vi "Reserve Session.vi"(6 "contextId":T4, 8 "error in":errorcluster, 9 "timeout (ms)":i32=-1, 10 "Request Data":T5, 11 "gRPC ID":T4) -> (0 "error out":errorcluster, 2 "Session Info":T1, 3 "gRPC ID out":T4)   [LabVIEW 2020]
uses:
  <vilib>/gRPC/LabVIEW gRPC Library/Shared/grpcId.ctl
  <vilib>/MeasurementLink/MeasurementLink Session Management Client/RPC Messages/ni_measurementlink_sessionmanagement_v1_ReserveSessionsRequest.ctl
  <vilib>/MeasurementLink/MeasurementLink Session Management Client/RPC Messages/ni_measurementlink_PinMapContext.ctl
  <vilib>/MeasurementLink/MeasurementLink Session Management Client/RPC Messages/ni_measurementlink_sessionmanagement_v1_SessionInformation.ctl
  <vilib>/MeasurementLink/MeasurementLink Session Management Client/RPC Messages/nidevice_grpc_Session.ctl
  <vilib>/MeasurementLink/MeasurementLink Session Management Client/RPC Messages/ni_measurementlink_sessionmanagement_v1_ChannelMapping.ctl
  <vilib>/MeasurementLink/MeasurementLink Session Management Client/MeasurementLink Session Management Client.lvlib
  <vilib>/gRPC/LabVIEW gRPC Library/grpc-lvsupport-release.lvlib
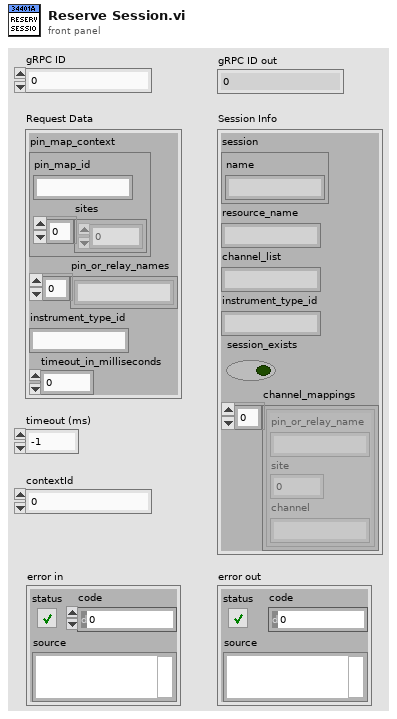
[diagram p1: front panel]
types:
  T1 = typedef "MeasurementLink Session Management Client.lvlib/ni_measurementlink_sessionmanagement_v1_SessionInformation.ctl" = cluster{"session":T2, "resource_name":string, "channel_list":string, "instrument_type_id":string, "session_exists":bool, "channel_mappings":T3[]}
  T2 = typedef "MeasurementLink Session Management Client.lvlib/nidevice_grpc_Session.ctl" = cluster{"name":string}
  T3 = typedef "MeasurementLink Session Management Client.lvlib/ni_measurementlink_sessionmanagement_v1_ChannelMapping.ctl" = cluster{"pin_or_relay_name":string, "site":i32, "channel":string}
  T4 = typedef "grpc-lvsupport-release.lvlib/grpcId.ctl" = u64
  T5 = typedef "MeasurementLink Session Management Client.lvlib/ni_measurementlink_sessionmanagement_v1_ReserveSessionsRequest.ctl" = cluster{"pin_map_context":T6, "pin_or_relay_names":string[], "instrument_type_id":string, "timeout_in_milliseconds":i32}
  T6 = typedef "MeasurementLink Session Management Client.lvlib/ni_measurementlink_PinMapContext.ctl" = cluster{"pin_map_id":string, "sites":i32[]}
  T7 = typedef "MeasurementLink Session Management Client.lvlib/ni_measurementlink_sessionmanagement_v1_ReserveSessionsResponse.ctl" = cluster{"sessions":T1[]}
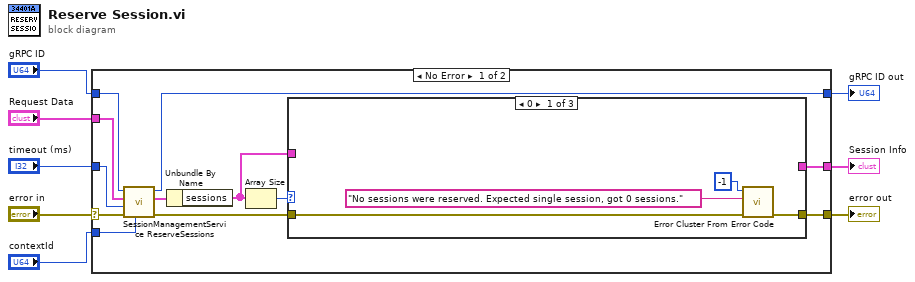
[diagram p0: block diagram]
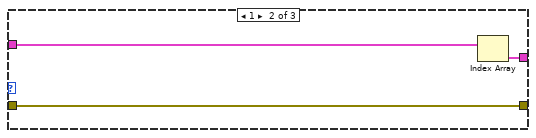
[diagram p2: hidden frame]
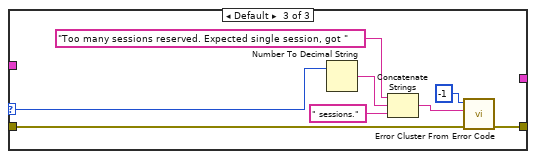
[diagram p3: hidden frame]
diagram:
  n1 = case shown="No Error" "error in" {
    selector: "error in" -> [w16 w36]
    tunnel: [w11 w36] -> w7
    tunnel: "gRPC ID" -> [w15 w37]
    tunnel: [w12 w37] -> w5
    tunnel: "Request Data" -> [w17 _]
    tunnel: "timeout (ms)" -> [w18 _]
    tunnel: "contextId" -> [w14 _]
    tunnel: [w9 _] -> w1
    frame No Error {
      n2 = call <vilib>:"SessionManagementService ReserveSessions.vi"("contextId"=w14, "error in"=w16, "timeout (ms)"=w18, "Request Data"=w17, "gRPC ID"=w15) -> ("error out"=w10:errorcluster, "Response Data"=w13:T7, "gRPC ID out"=w12:T4)  [unwired: 4 in]
      n3 = Unbundle By Name(w13) -> ("sessions"=w19:T1[])
      n4 = Array Size(array=w19) -> (size(s)=w20:i32)
      n5 = case shown="0" w20 {
        selector: w20 -> [_ _ w30]
        tunnel: w10 -> [w24 w25 w35]
        tunnel: [w21 w25 w33] -> w11
        tunnel: w19 -> [_ w27 _]
        tunnel: [_ w26 _] -> w9
        frame 0 {
          n6 = call <vilib>:"Error Cluster From Error Code.vi"("error in (no error)"=w24, "error message (\"\")"="No sessions were reserved. Expected single session, got 0 sessions." ("error message (\"\")"), "error code (0)"=-1) -> ("error out"=w21:errorcluster)  [unwired: 6 in]
        }
        frame 1 {
          n7 = Index Array(array=w27) -> (element=w26:T1)  [unwired: 1 in]
        }
        frame Default {
          n8 = Number To Decimal String(number=w30) -> (decimal integer string=w31:string)  [unwired: 1 in]
          n9 = Concatenate Strings("Too many sessions reserved. Expected single session, got " ("error message (\"\")"), w31, " sessions." ("string")) -> (w29:string)
          n10 = call <vilib>:"Error Cluster From Error Code.vi"("error in (no error)"=w35, "error message (\"\")"=w29, "error code (0)"=-1) -> ("error out"=w33:errorcluster)  [unwired: 6 in]
        }
      }
    }
    frame Error {
    }
  }
  "error out" <- w7
  "gRPC ID out" <- w5
  "Session Info" <- w1
